vi "Get_DT_Board_Info.vi"() -> (1 "DT Cluster Array":T1[](array[typedef]))   [LabVIEW 2017]
uses:
  Controls/DT_Cluster.ctl
  Controls/DT_Mode.ctl
  <userlib>/LV-Link3/PolySubVIs/DtCreateDinChan.vi
  <userlib>/LV-Link3/PolySubVIs/DtOLReadSingle.vi
  Globals/Meas_global.vi
panel:
  out "Array 6":i32[](array[numeric])
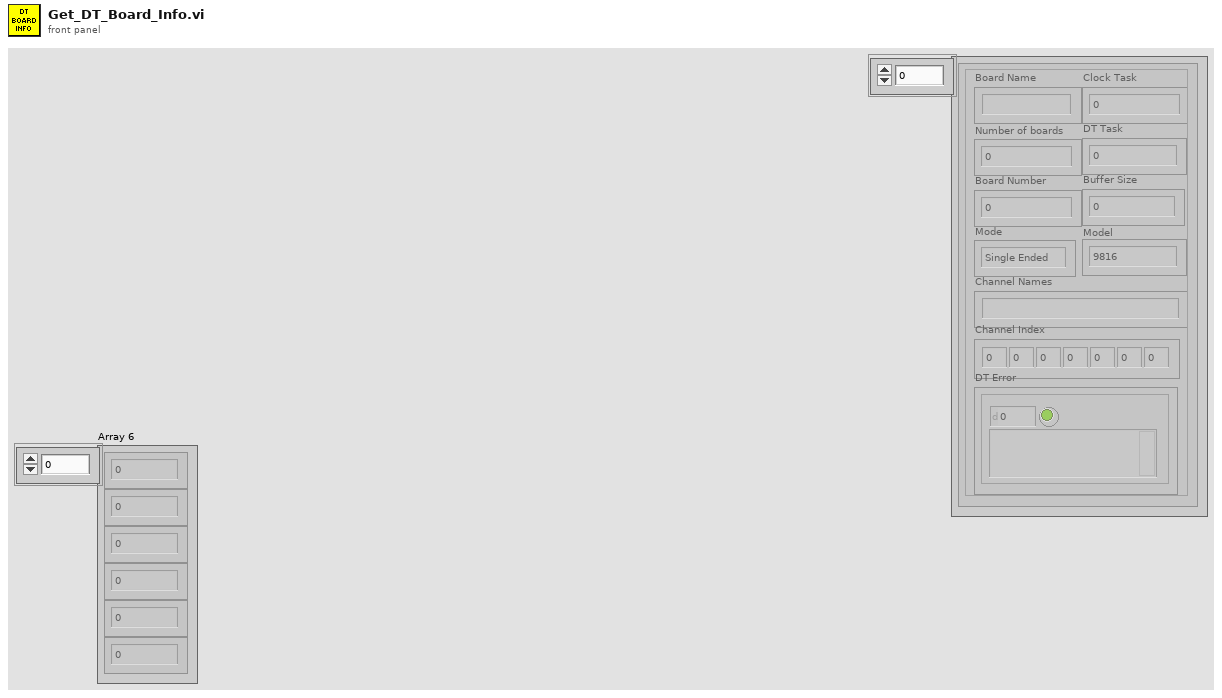
[diagram p1: front panel]
types:
  T1 = typedef "DT_Cluster.ctl" = cluster{"Board Name":string, "Number of boards":u32, "Board Number":u32, "Channel Names":string, "Channel Index":i32[], "DT Task":i32, "DT Error":errorcluster, "Mode":T2, "Buffer Size":u32, "Clock Task":i32, "Model":enum16{"9816", "9836", "9853"}}
  T2 = typedef "DT_Mode.ctl" = enum16{"Single Ended", "Differential"}
  T3 = typedef "Analysis_info_cluster.ctl" = cluster{"Colour":u32, "Inst type":T4, "Inst name":string, "Symbol":string, "Code name":string, "Extra Info":string, "Inst Array":T5, "Extra Titles":string[], "Extra Values":string[], "U":dbl, "u^2":dbl, "u^3":dbl, "u^4":dbl, "Skew_u":dbl, "Kurt_u":dbl, "Sd Error in Mean":dbl, "% u'/U":dbl, "X":dbl, "Y":dbl, "Z":dbl, "Timescale integral Estimate":dbl, "Sd Error in Variance":dbl, "Calib File":path, "Calib Constants":dbl[], "Output Position":bool, "Full Stats":bool, "Av Sampling Rate":dbl, "Av No of Samples":dbl, "Total Meas Time (s)":dbl, "ADAM Ch Name":string, "Max value":dbl, "Min value":dbl, "Req Sample Rate Hz":dbl, "Sync Delay Time (s)":dbl, "Ch No":i16, "Device ID":string, "Use Latest Calib":bool}
  T4 = typedef "Inst_type.ctl" = enum16{"Propeller anemometer", "Raw voltage", "Pressure Transducer", "Pitot-static tube", "Preston tube", "Hot wire", "Cross wire 1", "Cross wire 2", "Generic Linear", "Generic Polynomial", "Generic BackPoly", "Fast FID", "Thermocouple", "Cold wire", "Pulsed Wire", "LDA Vel", "LDA Tran time", "LDA Arr time", "Microphone"}
  T5 = typedef "Instrument_Array.ctl" = enum16{"PWA", "LDA", "Analogue"}
  T6 = cluster{"Board Number":u32, "Data Translation Board Cluster":T1}
  T7 = cluster{"Board Number":u32, "Data Translation Board Cluster":T1}[]
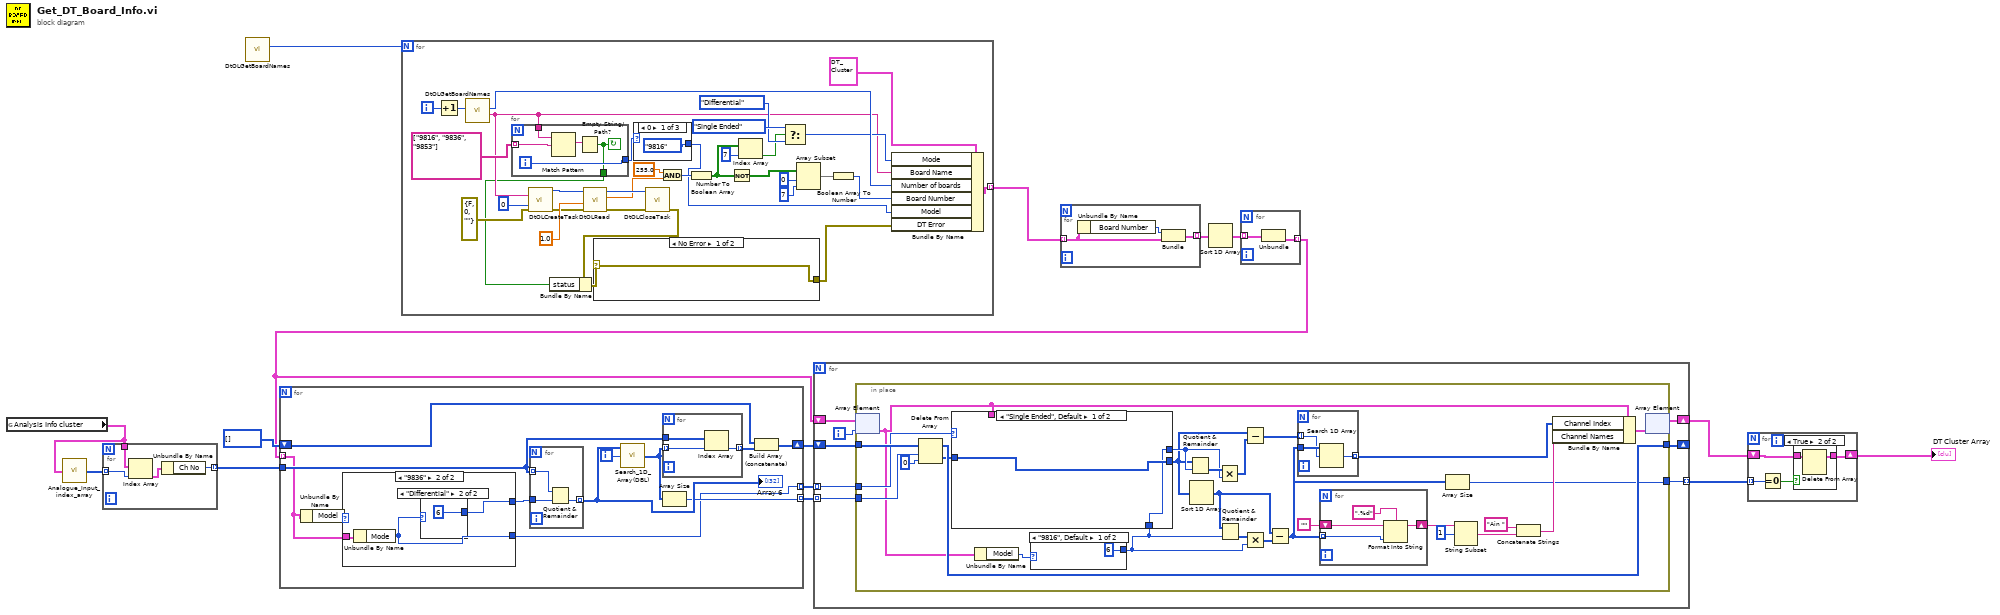
[diagram p0: block diagram]
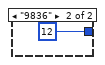
[diagram p3: hidden frame]
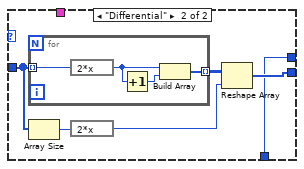
[diagram p4: hidden frame]
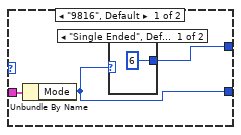
[diagram p5: hidden frame]
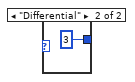
[diagram p6: hidden frame]
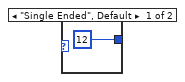
[diagram p7: hidden frame]
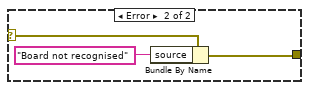
[diagram p8: hidden frame]
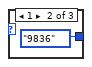
[diagram p9: hidden frame]
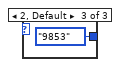
[diagram p10: hidden frame]
diagram:
  n1 = global read "Meas_global.vi" "Analysis Info cluster"() -> (w1:T3[])
  n2 = call "Analogue_Input_index_array.vi"("Analysis Info cluster"=w1) -> ("Array"=w2:i32[])
  n3 = for {
    tunnel: [w19] -> w8 mode=indexing
    tunnel: w2 -> [w18] mode=indexing
    tunnel: w1 -> [w17]
    n4 = Index Array(array=w17, index=w18) -> (element=w16:T3)
    n5 = Unbundle By Name(w16) -> ("Ch No"=w19:i16)
  }
  n6 = call <userlib>:"DtOLGetBoardNames.vi"() -> ("Number of boards"=w15:u32)  [unwired: 9 in, 2 out]
  n7 = for {
    N: w15 -> [_]
    tunnel: [w39] -> w14 mode=indexing
    i -> [w53]
    n8 = Increment(x=w53) -> (x+1=w52:i32)
    n9 = call <userlib>:"DtOLGetBoardNames.vi"("Select Board"=w52) -> ("Board Name"=w26:string, "Number of boards"=w42:u32)  [unwired: 8 in, 1 out]
    n10 = for {
      tunnel: string[] ["9816", "9836", "9853"] -> [w65] mode=indexing
      tunnel: w26 -> [w64]
      tunnel: [w62] -> w25
      tunnel: [w61] -> w22
      i -> [w62]
      stop <- w61 continue-if-true
      n11 = Match Pattern(string=w64, regular expression=w65) -> (match substring=w63:string)  [unwired: 1 in, 3 out]
      n12 = Empty String/Path?(string/path=w63) -> (empty?=w61:bool)
    }
    n13 = call-poly <userlib>:"DtOLCreateTask.vi"("Board Name"=w26, "Port Number"=u32 0, "error in (no error)"=errorcluster {"status"=FALSE, "code"=0, "source"=""} ("Error Out")) -> ("Task out"=w50:i32, "error out"=w47:errorcluster)  [unwired: 11 in]
    n14 = call-poly <userlib>:"DtOLRead.vi"("error in (no error)"=w47, "Timeout"=1.0 ("Samples Per Channel"), "Task in"=w50) -> ("error out"=w46:errorcluster, "Data Out"=w31:dbl, "Task out"=w45:i32)  [unwired: 6 in]
    n15 = case shown="0" w25 {
      tunnel: [enum16{"9816", "9836", "9853"}."9816" ("Model") enum16{"9816", "9836", "9853"}."9836" ("Model") enum16{"9816", "9836", "9853"}."9853" ("Model")] -> w24
      frame 0 {
      }
      frame 1 {
      }
      frame 2, Default {
      }
    }
    n16 = call <userlib>:"DtOLCloseTask.vi"("Error in"=w46, "Task in"=w45) -> ("Error Out"=w21:errorcluster)  [unwired: 9 in]
    n17 = Bundle By Name(cluster=w21, "status"=w22) -> (w23:errorcluster)
    n18 = case shown="No Error" w23 {
      selector: w23 -> [w54 w57]
      tunnel: [w54 w55] -> w20
      frame No Error {
      }
      frame Error {
        n19 = Bundle By Name(cluster=w57, "source"="Board not recognised") -> (w55:errorcluster)
      }
    }
    n20 = And(x=255.0, y=w31) -> (x .and. y?=w48:i32)
    n21 = Number To Boolean Array(number=w48) -> (Boolean array=w38:bool[])
    n22 = Not(x=w38) -> (.not. x?=w35:bool[])
    n23 = Index Array(array=w38, index=7) -> (element=w36:bool)
    n24 = Select(t=DT_Mode."Single Ended" ("Mode"), s=w36, f=DT_Mode."Differential") -> (s? t:f=w32:T2)
    n25 = Array Subset(array=w35, index=0, length=7) -> (w30:bool[])
    n26 = Boolean Array To Number(Boolean array=w30) -> (number=w28:u32)
    n27 = Bundle By Name(cluster=T1 {"Board Name"="", "Number of boards"=0, "Board Number"=0, "Channel Names"="", "Channel Index"=[], "DT Task"=0, "DT Error"={"status"=FALSE, "code"=0, "source"=""}, "Mode"=enum."Single Ended", "Buffer Size"=0, "Clock Task"=0, "Model"=enum."9816"} ("Data Translation Board Cluster"), "Mode"=w32, "Board Name"=w26, "Number of boards"=w42, "Board Number"=w28, "Model"=w24, "DT Error"=w20) -> (w39:T1)
  }
  n28 = for {
    tunnel: w14 -> [w68] mode=indexing
    tunnel: [w66] -> w13 mode=indexing
    n29 = Unbundle By Name(w68) -> ("Board Number"=w67:u32)
    n30 = Bundle("Board Number"=w67, "Data Translation Board Cluster"=w68) -> (w66:T6)  [unwired: 1 in]
  }
  n31 = Sort 1D Array(array=w13) -> (sorted array=w12:T7)
  n32 = for {
    tunnel: w12 -> [w70] mode=indexing
    tunnel: [w69] -> w6 mode=indexing
    n33 = Unbundle(w70) -> ("Data Translation Board Cluster"=w69:T1)  [unwired: 1 out]
  }
  n34 = for {
    tunnel: w8 -> [w75]
    tunnel: [w79] -> w11 mode=indexing
    shift-right: [w77] -> w9
    shift-left: i32[] [] -> [w76]
    tunnel: w6 -> [w72] mode=indexing
    tunnel: [w73] -> w7 mode=indexing
    i -> [w82]
    n35 = Unbundle By Name(w72) -> ("Model"=w71:enum16{"9816", "9836", "9853"})
    n36 = case shown="\"9836\"" w71 {
      tunnel: [w85 w90] -> w74
      tunnel: w72 -> [w84 w89]
      tunnel: [w83 w88] -> w73
      frame "9816", Default {
        n37 = Unbundle By Name(w84) -> ("Mode"=w83:T2)
        n38 = case shown="\"Single Ended\", Default" w83 {
          tunnel: [6 ("y") 3 ("y")] -> w85
          frame "Single Ended", Default {
          }
          frame "Differential" {
          }
        }
      }
      frame "9836" {
        n39 = Unbundle By Name(w89) -> ("Mode"=w88:T2)
        n40 = case shown="\"Differential\"" w88 {
          tunnel: [12 ("y") 6 ("y")] -> w90
          frame "Single Ended", Default {
          }
          frame "Differential" {
          }
        }
      }
    }
    n41 = for {
      tunnel: w75 -> [w97] mode=indexing
      tunnel: [w98] -> w81 mode=indexing
      tunnel: w74 -> [w96]
      n42 = Quotient & Remainder(x=w97, y=w96) -> (floor(x/y)=w98:i32)  [unwired: 1 out]
    }
    "Array 6" <- w81
    n43 = call "Search_1D_Array(DBL).vi"("Array"=w81, "Element Data"=w82) -> ("Indicies of Elements"=w80:i32[])  [unwired: 6 in, 1 out]
    n44 = for {
      tunnel: w80 -> [w94] mode=indexing
      tunnel: w75 -> [w95]
      tunnel: [w93] -> w78 mode=indexing
      n45 = Index Array(array=w95, index=w94) -> (element=w93:i16)
    }
    n46 = Array Size(array=w80) -> (size(s)=w79:i32)
    n47 = Build Array (concatenate)(w76, w78) -> (w77:i32[])
  }
  n48 = for {
    tunnel: w11 -> [w105] mode=indexing
    shift-right: [w104] -> _
    shift-left: w9 -> [w106]
    shift-right: [w101] -> w4
    shift-left: w6 -> [w102]
    tunnel: w7 -> [w103] mode=indexing
    tunnel: [w99] -> w5 mode=indexing
    i -> [w100]
    n49 = in-place {
      in-place-border: w106 -> [w133]
      in-place-border: w105 -> [w132]
      in-place-border: [w126] -> w104
      in-place-border: w103 -> [w115]
      in-place-border: [w110] -> w99
      n50 = in-place-array #1(w102, w100) -> (w108:T1)
      n51 = Delete From Array(array=w133, length=w132, index=0) -> (deleted portion=w124:i32[], array with subset deleted=w126:i32[])
      n52 = Unbundle By Name(w108) -> ("Model"=w109:enum16{"9816", "9836", "9853"})
      n53 = case shown="\"9816\", Default" w109 {
        tunnel: [6 ("offset (0)") 12 ("offset (0)")] -> w107
        frame "9816", Default {
        }
        frame "9836" {
        }
      }
      n54 = case shown="\"Single Ended\", Default" w115 {
        tunnel: w124 -> [w137 w140]
        tunnel: [w136 w138] -> w118
        tunnel: [w137 w139] -> w116
        tunnel: w108 -> [_ _]
        tunnel: w107 -> [w136 w138]
        frame "Single Ended", Default {
        }
        frame "Differential" {
          n55 = for {
            tunnel: [w146] -> w142 mode=indexing
            tunnel: w140 -> [w144] mode=indexing
            n56 = expression code="2*x"(w144) -> (w145:i32)
            n57 = Increment(x=w145) -> (x+1=w147:i32)
            n58 = Build Array(w145, w147) -> (w146:i32[])
          }
          n59 = Array Size(array=w140) -> (size(s)=w143:i32)
          n60 = expression code="2*x"(w143) -> (w141:i32)
          n61 = Reshape Array(w142, w141) -> (w139:i32[])
        }
      }
      n62 = Quotient & Remainder(x=w116, y=w118) -> (floor(x/y)=w120:i32[])  [unwired: 1 out]
      n63 = Sort 1D Array(array=w116) -> (sorted array=w121:i32[])
      n64 = Multiply(x=w120, y=w118) -> (x*y=w119:i32[])
      n65 = Quotient & Remainder(x=w121, y=w107) -> (floor(x/y)=w122:i32[])  [unwired: 1 out]
      n66 = Subtract(x=w116, y=w119) -> (x-y=w117:i32[])
      n67 = Multiply(x=w122, y=w107) -> (x*y=w123:i32[])
      n68 = Subtract(x=w121, y=w123) -> (x-y=w111:i32[])
      n69 = for {
        tunnel: w111 -> [w154]
        tunnel: w117 -> [w153] mode=indexing
        tunnel: [w152] -> w113 mode=indexing
        n70 = Search 1D Array(1D array=w154, element=w153) -> (index of element=w152:i32)  [unwired: 1 in]
      }
      n71 = for {
        shift-right: [w149] -> w131
        shift-left: "" -> [w150]
        tunnel: w111 -> [w148] mode=indexing
        n72 = Format Into String(format string=",%d", initial string=w150, w148) -> (resulting string=w149:string)  [unwired: 1 in, 1 out]
      }
      n73 = Array Size(array=w111) -> (size(s)=w110:i32)
      n74 = String Subset(string=w131, offset (0)=1) -> (substring=w128:string)  [unwired: 1 in]
      n75 = Concatenate Strings("Ain ", w128) -> (w112:string)
      n76 = Bundle By Name(cluster=w108, "Channel Index"=w113, "Channel Names"=w112) -> (w114:T1)
      n77 = in-place-array #1(w114) -> (w101:T1[])  [unwired: 1 out]
    }
  }
  n78 = for {
    tunnel: w5 -> [w158] mode=indexing
    shift-right: [w155] -> w3
    shift-left: w4 -> [w157]
    n79 = Equal To 0?(x=w158) -> (x = 0?=w156:bool)
    n80 = case shown="True" w156 {
      tunnel: w157 -> [w159 w161]
      tunnel: [w159 w160] -> w155
      frame False {
      }
      frame True {
        n81 = Delete From Array(array=w161) -> (array with subset deleted=w160:T1[])  [unwired: 2 in, 1 out]
      }
    }
  }
  "DT Cluster Array" <- w3
